vi "Handle Error.vi"(8 "error in (no error)":errorcluster caption="错误输入（无错误）", 11 "THM-V6数字型温湿度 in":refnum<class "THM-V6数字型温湿度.lvclass"> caption="操作者输入") -> (0 "error out":errorcluster caption="错误输出", 2 "stop actor?":bool=TRUE caption="停止操作者？", 3 "THM-V6数字型温湿度 out":refnum<class "THM-V6数字型温湿度.lvclass"> caption="操作者输出")   [LabVIEW 2016, in "THM-V6数字型温湿度.lvlib" / "THM-V6数字型温湿度.lvclass"]
doc: "(<B>Filename</B>: Actor Framework.lvlib:Actor.lvclass:Handle Error.vi)\n\nDefines how the actor handles an error that occurred while processing a message.默认情况下，该方法不执行任何操作，仅停止操作者。"
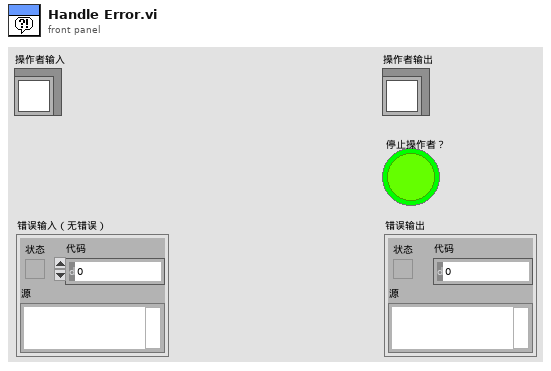
[diagram p1: front panel]
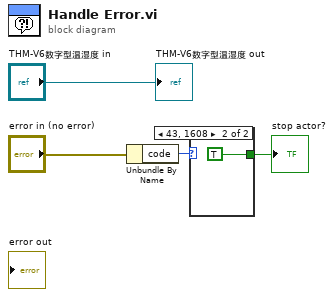
[diagram p0: block diagram]
diagram:
  n1 = Unbundle By Name("error in (no error)") -> ("code"=w4:i32)
  n2 = case shown="43, 1608" w4 {
    tunnel: [_ TRUE] -> w3
    frame 0, Default {
    }
    frame 43, 1608 {
    }
  }
  "stop actor?" <- w3
  "THM-V6数字型温湿度 out" <- "THM-V6数字型温湿度 in"
